vi "Raman Spectrum Import Control.vi"(6 "Iterations":i32, 7 "Collect Spectra?":bool, 9 "counter in":i32, 10 "Filename array in":string[][](array[string]), 11 "Filepath cluster in":T1) -> (0 "Filename array out":string[][](array[string]), 1 "Filepath cluster out 2":T1, 2 "Filepath Cluster out":T1, 3 "Spectra Array":cluster{i32[], i32[]}[](array[cluster]), 4 "counter out":i32, 5 "Display Spectra?":bool)   [LabVIEW 2015]
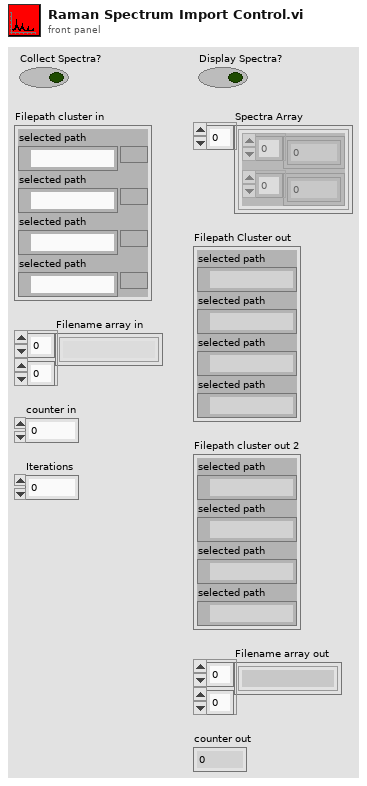
[diagram p1: front panel]
types:
  T1 = cluster{"selected path":path, "selected path":path, "selected path":path, "selected path":path}
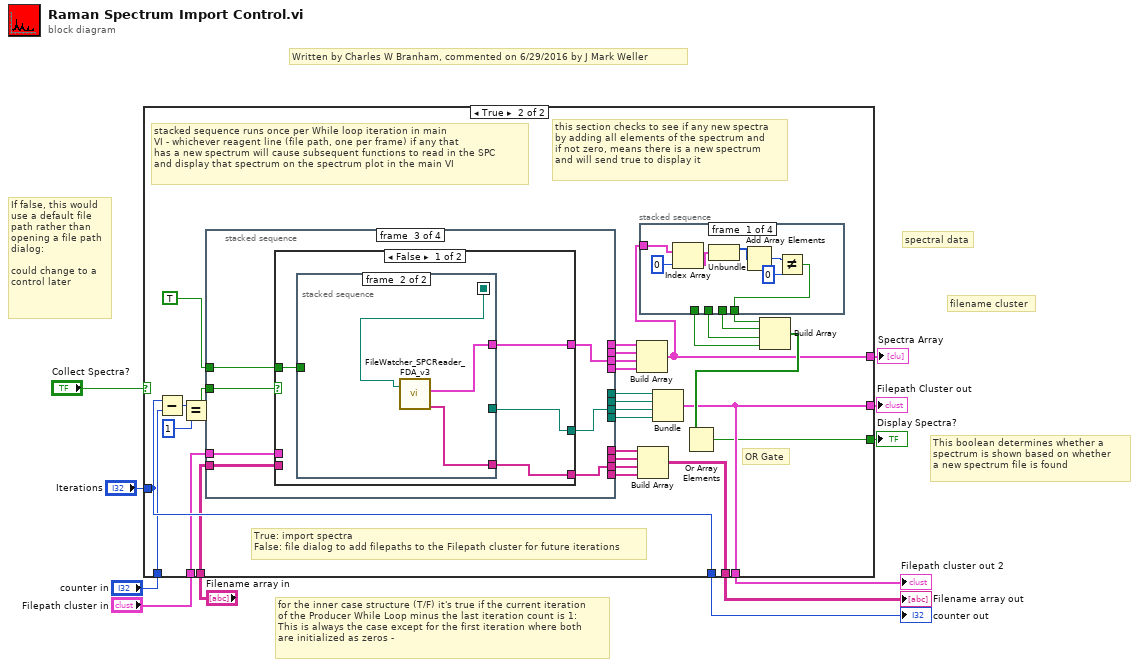
[diagram p0: block diagram]
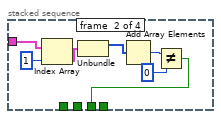
[diagram p3: hidden frame]
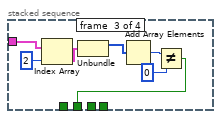
[diagram p4: hidden frame]
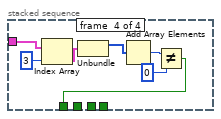
[diagram p5: hidden frame]
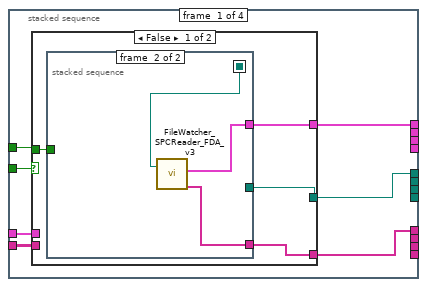
[diagram p6: hidden frame]
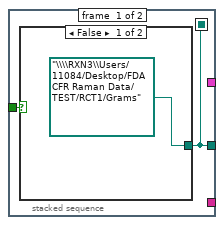
[diagram p7: hidden frame]
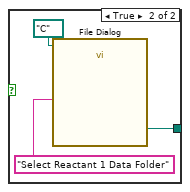
[diagram p8: hidden frame]
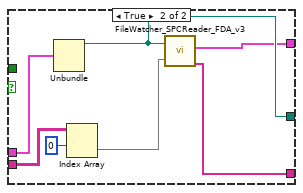
[diagram p9: hidden frame]
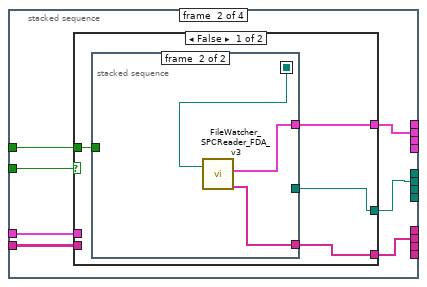
[diagram p10: hidden frame]
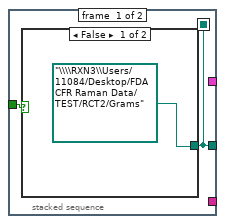
[diagram p11: hidden frame]
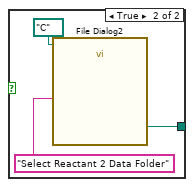
[diagram p12: hidden frame]
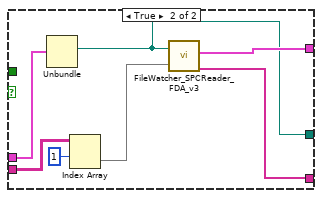
[diagram p13: hidden frame]
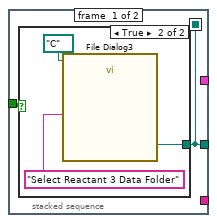
[diagram p14: hidden frame]
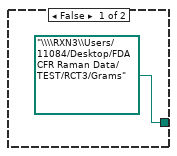
[diagram p15: hidden frame]
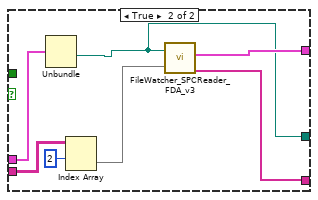
[diagram p16: hidden frame]
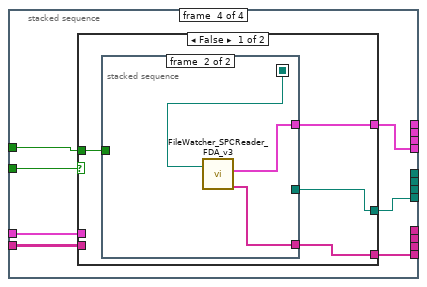
[diagram p17: hidden frame]
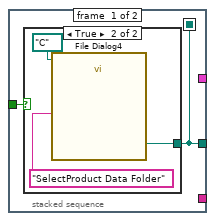
[diagram p18: hidden frame]
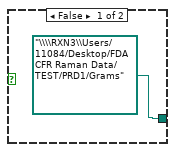
[diagram p19: hidden frame]
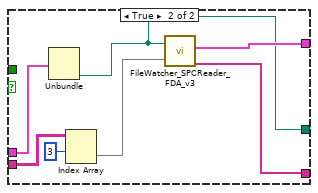
[diagram p20: hidden frame]
diagram:
  # "If false, this would\nuse a default file\npath rather than \nopening a file path\ndialog:\n\ncould change to a\ncontrol later"
  # "Written by Charles W Branham, commented on 6/29/2016 by J Mark Weller"
  # "filename cluster"
  # "spectral data"
  # "This boolean determines whether a\nspectrum is shown based on whether\na new spectrum file is found"
  # "for the inner case structure (T/F) it's true if the current iteration\nof the Producer While Loop minus the last iteration count is 1:\nThis is always the case except for the first iteration where both\nare initialized as zeros -"
  n1 = case shown="True" "Collect Spectra?" {
    tunnel: "counter in" -> [_ w36]
    tunnel: [_ w37] -> w3
    tunnel: "Iterations" -> [_ w37]
    tunnel: [_ w12] -> w11
    tunnel: [_ w14] -> w5
    tunnel: "Filepath cluster in" -> [_ w35]
    tunnel: [_ w31] -> w7
    tunnel: "Filename array in" -> [_ w34]
    tunnel: [_ w14] -> w9
    tunnel: [_ w13] -> w10
    frame False {
      # "Not importing Raman spectra from the RXN4 computer"
    }
    frame True {
      # "True: import spectra\nFalse: file dialog to add filepaths to the Filepath cluster for future iterations"
      # "stacked sequence runs once per While loop iteration in main\nVI - whichever reagent line (file path, one per frame) if any that\nhas a new spectrum will cause subsequent functions to read in the SPC\nand display that spectrum on the spectrum plot in the main VI"
      # "OR Gate"
      # "this section checks to see if any new spectra\nby adding all elements of the spectrum and\nif not zero, means there is a new spectrum\nand will send true to display it"
      n2 = Subtract(x=w37, y=w36) -> (x-y=w40:i32)
      n3 = Equal?(x=w40, y=1) -> (x = y?=w38:bool)
      n4 = stacked-sequence {
        tunnel: w38 -> [w75 w102 w129 w156]
        tunnel: [w70 _ _ _] -> w24
        tunnel: w35 -> [w74 w101 w128 w155]
        tunnel: [w73 _ _ _] -> w32
        tunnel: w34 -> [w72 w100 w127 w154]
        tunnel: [w71 _ _ _] -> w25
        tunnel: [_ w99 _ _] -> w33
        tunnel: [_ w97 _ _] -> w23
        tunnel: [_ w98 _ _] -> w30
        tunnel: [_ _ w126 _] -> w29
        tunnel: [_ _ w124 _] -> w22
        tunnel: [_ _ w125 _] -> w28
        tunnel: [_ _ _ w153] -> w27
        tunnel: [_ _ _ w151] -> w21
        tunnel: [_ _ _ w152] -> w26
        tunnel: TRUE ("Default File Path or Specify? (T = specify)") -> [w69 w96 w123 w150]
        frame #0 {
          n5 = case shown="False" w75 {
            tunnel: [w79 w90] -> w71
            tunnel: [w77 w91] -> w70
            tunnel: [w78 w89] -> w73
            tunnel: w74 -> [_ w93]
            tunnel: w72 -> [_ w95]
            tunnel: w69 -> [w76 _]
            frame False {
              n6 = stacked-sequence {
                seq-local: [w80 _] -> [_ w86]
                tunnel: [w80 _] -> w77
                tunnel: [_ w88] -> w79
                tunnel: [_ w87] -> w78
                tunnel: w76 -> [w81 _]
                frame #0 {
                  n7 = case shown="False" w81 {
                    tunnel: [path "\\\\RXN3\\Users/11084/Desktop/FDA CFR Raman Data/TEST/RCT1/Grams" ("start path") w84] -> w80
                    frame False {
                    }
                    frame True {
                      n8 = call "File Dialog"("start path"=path "C:/", "prompt"="Select Reactant 1 Data Folder") -> ("selected path"=w84:path)  [unwired: 10 in, 3 out]
                    }
                  }
                }
                frame #1 {
                  n9 = call "FileWatcher_SPCReader_FDA_v3.vi"("appended path"=w86) -> ("Filesnames out"=w87:string[], "Raman Spectrum"=w88:cluster{i32[], i32[]})  [unwired: 2 in, 2 out]
                }
              }
            }
            frame True {
              n10 = Unbundle(w93) -> ("selected path"=w91:path)  [unwired: 3 out]
              n11 = Index Array(array=w95, index (row)=0) -> (element=w92:string[])  [unwired: 1 in]
              n12 = call "FileWatcher_SPCReader_FDA_v3.vi"("Filenames in"=w92, "appended path"=w91) -> ("Filesnames out"=w89:string[], "Raman Spectrum"=w90:cluster{i32[], i32[]})  [unwired: 1 in, 2 out]
            }
          }
        }
        frame #1 {
          n13 = case shown="False" w102 {
            tunnel: [w106 w122] -> w99
            tunnel: [w104 w117] -> w97
            tunnel: [w105 w121] -> w98
            tunnel: w101 -> [_ w116]
            tunnel: w100 -> [_ w119]
            tunnel: w96 -> [w103 _]
            frame False {
              n14 = stacked-sequence {
                seq-local: [w107 _] -> [_ w113]
                tunnel: [w107 _] -> w104
                tunnel: [_ w115] -> w106
                tunnel: [_ w114] -> w105
                tunnel: w103 -> [w108 _]
                frame #0 {
                  n15 = case shown="False" w108 {
                    tunnel: [path "\\\\RXN3\\Users/11084/Desktop/FDA CFR Raman Data/TEST/RCT2/Grams" ("start path") w111] -> w107
                    frame False {
                    }
                    frame True {
                      n16 = call "File Dialog2"("start path"=path "C:/", "prompt"="Select Reactant 2 Data Folder") -> ("selected path"=w111:path)  [unwired: 10 in, 3 out]
                    }
                  }
                }
                frame #1 {
                  n17 = call "FileWatcher_SPCReader_FDA_v3.vi"("appended path"=w113) -> ("Filesnames out"=w114:string[], "Raman Spectrum"=w115:cluster{i32[], i32[]})  [unwired: 2 in, 2 out]
                }
              }
            }
            frame True {
              n18 = Unbundle(w116) -> ("selected path"=w117:path)  [unwired: 3 out]
              n19 = Index Array(array=w119, index (row)=1) -> (element=w118:string[])  [unwired: 1 in]
              n20 = call "FileWatcher_SPCReader_FDA_v3.vi"("Filenames in"=w118, "appended path"=w117) -> ("Filesnames out"=w121:string[], "Raman Spectrum"=w122:cluster{i32[], i32[]})  [unwired: 1 in, 2 out]
            }
          }
        }
        frame #2 {
          n21 = case shown="False" w129 {
            tunnel: [w133 w149] -> w126
            tunnel: [w131 w143] -> w124
            tunnel: [w132 w148] -> w125
            tunnel: w128 -> [_ w144]
            tunnel: w127 -> [_ w146]
            tunnel: w123 -> [w130 _]
            frame False {
              n22 = stacked-sequence {
                seq-local: [w134 _] -> [_ w140]
                tunnel: [w134 _] -> w131
                tunnel: [_ w142] -> w133
                tunnel: [_ w141] -> w132
                tunnel: w130 -> [w135 _]
                frame #0 {
                  n23 = case shown="True" w135 {
                    tunnel: [path "\\\\RXN3\\Users/11084/Desktop/FDA CFR Raman Data/TEST/RCT3/Grams" ("start path") w138] -> w134
                    frame False {
                    }
                    frame True {
                      n24 = call "File Dialog3"("start path"=path "C:/", "prompt"="Select Reactant 3 Data Folder") -> ("selected path"=w138:path)  [unwired: 10 in, 3 out]
                    }
                  }
                }
                frame #1 {
                  n25 = call "FileWatcher_SPCReader_FDA_v3.vi"("appended path"=w140) -> ("Filesnames out"=w141:string[], "Raman Spectrum"=w142:cluster{i32[], i32[]})  [unwired: 2 in, 2 out]
                }
              }
            }
            frame True {
              n26 = Unbundle(w144) -> ("selected path"=w143:path)  [unwired: 3 out]
              n27 = Index Array(array=w146, index (row)=2) -> (element=w145:string[])  [unwired: 1 in]
              n28 = call "FileWatcher_SPCReader_FDA_v3.vi"("Filenames in"=w145, "appended path"=w143) -> ("Filesnames out"=w148:string[], "Raman Spectrum"=w149:cluster{i32[], i32[]})  [unwired: 1 in, 2 out]
            }
          }
        }
        frame #3 {
          n29 = case shown="False" w156 {
            tunnel: [w160 w176] -> w153
            tunnel: [w158 w170] -> w151
            tunnel: [w159 w175] -> w152
            tunnel: w155 -> [_ w171]
            tunnel: w154 -> [_ w173]
            tunnel: w150 -> [w157 _]
            frame False {
              n30 = stacked-sequence {
                seq-local: [w161 _] -> [_ w167]
                tunnel: [w161 _] -> w158
                tunnel: [_ w169] -> w160
                tunnel: [_ w168] -> w159
                tunnel: w157 -> [w162 _]
                frame #0 {
                  n31 = case shown="True" w162 {
                    tunnel: [path "\\\\RXN3\\Users/11084/Desktop/FDA CFR Raman Data/TEST/PRD1/Grams" ("start path") w165] -> w161
                    frame False {
                    }
                    frame True {
                      n32 = call "File Dialog4"("start path"=path "C:/", "prompt"="SelectProduct Data Folder") -> ("selected path"=w165:path)  [unwired: 10 in, 3 out]
                    }
                  }
                }
                frame #1 {
                  n33 = call "FileWatcher_SPCReader_FDA_v3.vi"("appended path"=w167) -> ("Filesnames out"=w168:string[], "Raman Spectrum"=w169:cluster{i32[], i32[]})  [unwired: 2 in, 2 out]
                }
              }
            }
            frame True {
              n34 = Unbundle(w171) -> ("selected path"=w170:path)  [unwired: 3 out]
              n35 = Index Array(array=w173, index (row)=3) -> (element=w172:string[])  [unwired: 1 in]
              n36 = call "FileWatcher_SPCReader_FDA_v3.vi"("Filenames in"=w172, "appended path"=w170) -> ("Filesnames out"=w175:string[], "Raman Spectrum"=w176:cluster{i32[], i32[]})  [unwired: 1 in, 2 out]
            }
          }
        }
      }
      n37 = Build Array(w25, w33, w29, w27) -> (w12:cluster{i32[], i32[]}[])
      n38 = Build Array(w32, w30, w28, w26) -> (w31:string[][])
      n39 = stacked-sequence {
        tunnel: w12 -> [w45 w52 w59 w66]
        tunnel: [w41 _ _ _] -> w20
        tunnel: [_ w48 _ _] -> w19
        tunnel: [_ _ w55 _] -> w18
        tunnel: [_ _ _ w62] -> w17
        frame #0 {
          n40 = Index Array(array=w45, index=0) -> (element=w44:cluster{i32[], i32[]})
          n41 = Unbundle(w44) -> (w43:i32[])  [unwired: 1 out]
          n42 = Add Array Elements(numeric array=w43) -> (sum=w46:i32)
          n43 = Not Equal?(x=w46, y=0) -> (x != y?=w41:bool)
        }
        frame #1 {
          n44 = Index Array(array=w52, index=1) -> (element=w51:cluster{i32[], i32[]})
          n45 = Unbundle(w51) -> (w50:i32[])  [unwired: 1 out]
          n46 = Add Array Elements(numeric array=w50) -> (sum=w53:i32)
          n47 = Not Equal?(x=w53, y=0) -> (x != y?=w48:bool)
        }
        frame #2 {
          n48 = Index Array(array=w59, index=2) -> (element=w58:cluster{i32[], i32[]})
          n49 = Unbundle(w58) -> (w57:i32[])  [unwired: 1 out]
          n50 = Add Array Elements(numeric array=w57) -> (sum=w60:i32)
          n51 = Not Equal?(x=w60, y=0) -> (x != y?=w55:bool)
        }
        frame #3 {
          n52 = Index Array(array=w66, index=3) -> (element=w65:cluster{i32[], i32[]})
          n53 = Unbundle(w65) -> (w64:i32[])  [unwired: 1 out]
          n54 = Add Array Elements(numeric array=w64) -> (sum=w67:i32)
          n55 = Not Equal?(x=w67, y=0) -> (x != y?=w62:bool)
        }
      }
      n56 = Bundle("selected path"=w24, "selected path"=w23, "selected path"=w22, "selected path"=w21) -> (w14:T1)  [unwired: 1 in]
      n57 = Build Array(w20, w19, w18, w17) -> (w16:bool[])
      n58 = Or Array Elements(Boolean array=w16) -> (logical OR=w13:bool)
    }
  }
  "Spectra Array" <- w11
  "Display Spectra?" <- w10
  "Filepath Cluster out" <- w9
  "Filename array out" <- w7
  "Filepath cluster out 2" <- w5
  "counter out" <- w3
